vi "WPI_ERRSolenoidAllocation.vi"(8 "error in (no error)":errorcluster, 10 "SolenoidChannel":T1=enum."Solenoid 1") -> (0 "ERRSolenoidAllocation":errorcluster)   [LabVIEW 2017]
doc: "This software is licensed. Open the labview\\readme\\WPI Robotics Library Open Source License.txt file for more information."
uses:
  <vilib>/Rock Robotics/WPI/Solenoid/WPI_SolenoidChannel.ctl
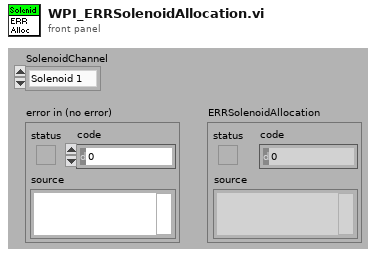
[diagram p1: front panel]
types:
  T1 = typedef "WPI_SolenoidChannel.ctl" = enum8{"Solenoid 0", "Solenoid 1", "Solenoid 2", "Solenoid 3", "Solenoid 4", "Solenoid 5", "Solenoid 6", "Solenoid 7", "Invalid"}
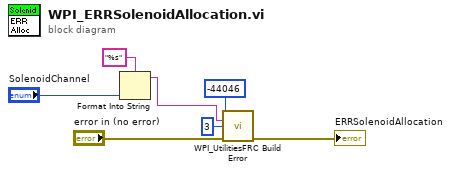
[diagram p0: block diagram]
diagram:
  n1 = Format Into String(format string="%s", "SolenoidChannel") -> (resulting string=w2:string)  [unwired: 2 in, 1 out]
  n2 = call <vilib>:"WPI_UtilitiesFRC Build Error.vi"("error code"=-44046 ("code"), "extra error text"=w2, "chain levels to remove (1)"=3, "error in (no error)"="error in (no error)") -> ("error out"=→"ERRSolenoidAllocation":errorcluster)  [unwired: 1 in, 10 out]
